vi "microFPGA_init.vi"(8 "error in (no error)":errorcluster) -> (0 "error out":errorcluster, 3 "VISA resource name out":refnum<visa-resource-name>="COM118")   [LabVIEW 2021]
uses:
  <vilib>/Instr/_visa.llb/VISA Open Access Mode.ctl
  <vilib>/Instr/_visa.llb/VISA Configure Serial Port (Instr).vi
panel:
  in  "stop":bool=TRUE
  in  "Termination Character":u8=10 format="%.0x"
  in  "VISA resource name":refnum<visa-resource-name>="COM118"
  in  "End Read on Termination Character?":bool
  # "choose the COM port"
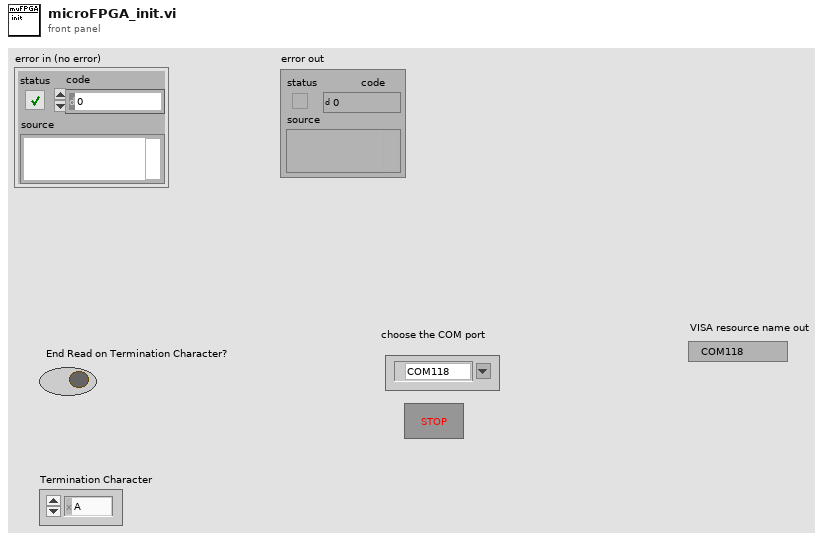
[diagram p1: front panel]
types:
  T1 = cluster{"baud rate":u32, "data bits":u16, "parity":enum16{"None", "Odd", "Even", "Mark", "Space"}, "stop bits":u16, "flow control":u16}
  T2 = typedef "VISA Open Access Mode.ctl" = u32
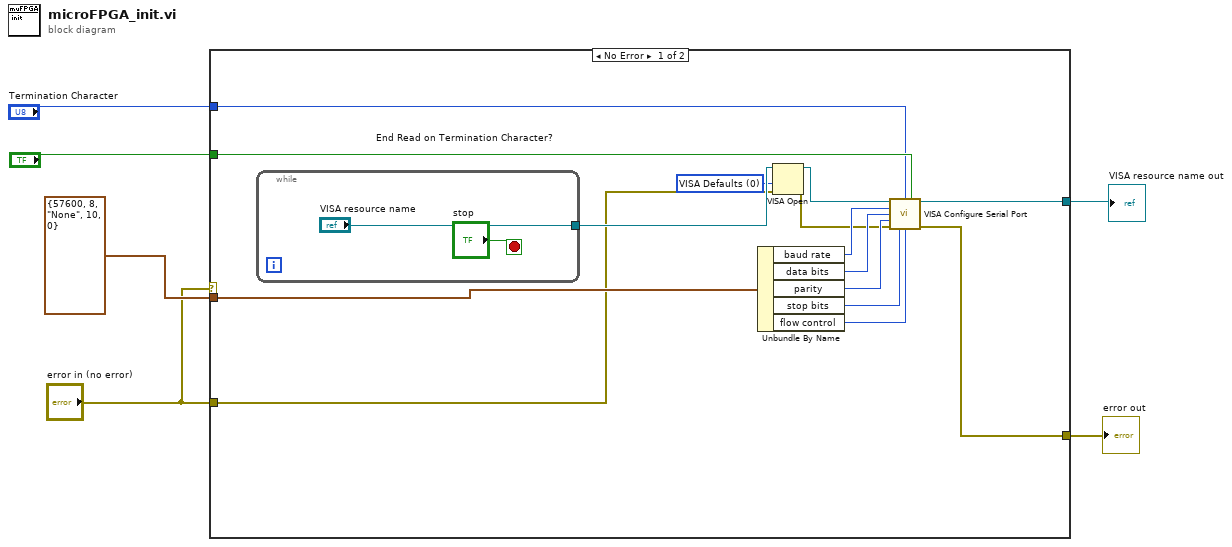
[diagram p0: block diagram]
diagram:
  n1 = case shown="No Error" "error in (no error)" {
    tunnel: T1 {"baud rate"=57600, "data bits"=8, "parity"=enum."None", "stop bits"=10, "flow control"=0} ("Serial Settings") -> [w18 _]
    tunnel: "End Read on Termination Character?" -> [w17 _]
    tunnel: "Termination Character" -> [w15 _]
    tunnel: "error in (no error)" -> [w10 w24]
    tunnel: [w8 w24] -> w3
    tunnel: [w7 _] -> w1
    frame No Error {
      w13 = T2 0 items=["VISA Defaults"=0, "Exclusive Lock"=1, "Load Configured Settings"=4] ("Access Mode")
      n2 = while {
        tunnel: ["VISA resource name"] -> w14
        stop <- "stop" stop-if-true
      }
      n3 = Unbundle By Name(w18) -> ("baud rate"=w11:u32, "data bits"=w19:u16, "parity"=w20:enum16{"None", "Odd", "Even", "Mark", "Space"}, "stop bits"=w21:u16, "flow control"=w16:u16)
      n4 = VISA Open(access mode=w13, error in (no error)=w10, VISA resource name=w14) -> (VISA resource name=w12:refnum<visa-resource-name>, error out=w9:errorcluster)  [unwired: 2 in]
      n5 = call-poly "VISA Configure Serial Port"("VISA resource name"=w12, "termination char\n(0xA = '\\n' = LF)"=w15, "Enable Termination\nChar (T)"=w17, "baud rate (9600)"=w11, "data bits (8)"=w19, "parity (0:none)"=w20, "error in (no error)"=w9, "stop bits (10: 1 bit)"=w21, "flow control (0:none)"=w16) -> ("VISA resource name out"=w7:refnum<visa-resource-name>, "error out"=w8:errorcluster)  [unwired: 1 in, 4 out]
    }
    frame Error {
    }
  }
  "error out" <- w3
  "VISA resource name out" <- w1
